vi "Configure TS Panel.vi"(8 "error in":errorcluster, 11 "DeepU Test Stand in":refnum<class "DeepU Test Stand.lvclass">) -> (0 "error out":errorcluster, 3 "DeepU Test Stand out":refnum<class "DeepU Test Stand.lvclass">)   [LabVIEW 2019, in "Test Stands.lvlib" / "DeepU Test Stand.lvclass"]
uses:
  DeepU Test Stand.lvclass
  C:/Users/wg/Documents/LV_Projects/test-stand/App/Generic Test Stand/Generic Test Stand.lvclass
  Generic Test Stand/Generic Test Stand.lvclass/Generic Test Stand.ctl
  DeepU Test Stand.lvclass/DeepU Test Stand.ctl
  Generic Test Stand/Generic Test Stand.lvclass
  Results/DeepU Results/DeepU Front Panel.vi
  Results/DeepU Results/DeepU Results.lvclass
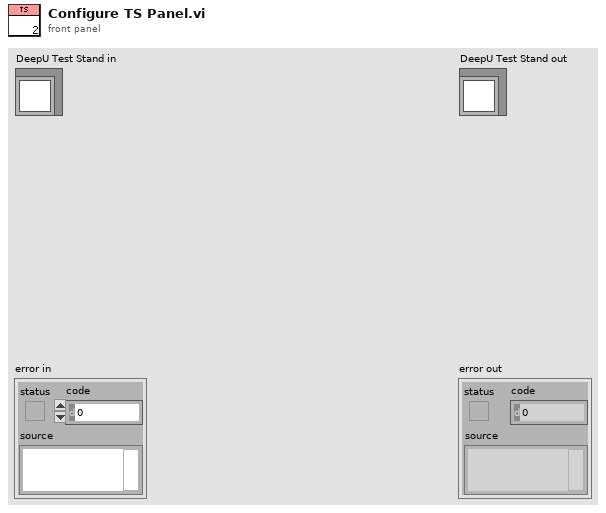
[diagram p1: front panel]
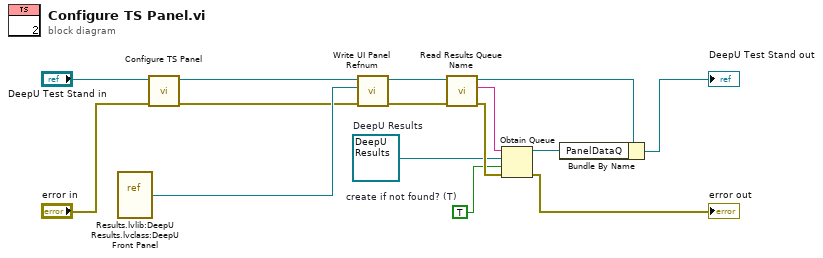
[diagram p0: block diagram]
diagram:
  w2 = refnum<class "DeepU Results.lvclass"> refnum  # DeepU Results
  w4 = TRUE  # create if not found? (T)
  n1 = vi-ref "Results.lvlib:DeepU Results.lvclass:DeepU Front Panel.vi"() -> (w15:refnum<vi>)
  n2 = call-parent "Configure TS Panel.vi"("error in (no error)"="error in", "Generic Test Stand in"="DeepU Test Stand in") -> ("error out"=w11:errorcluster, "Generic Test Stand out"=w13:refnum<class "DeepU Test Stand.lvclass">)  [unwired: 8 in]
  n3 = call "Write UI Panel Refnum.vi"("error in (no error)"=w11, "UI Panel Refnum"=w15, "Generic Test Stand in"=w13) -> ("error out"=w7:errorcluster, "Generic Test Stand out"=w10:refnum<class "DeepU Test Stand.lvclass">)  [unwired: 7 in]
  n4 = call "Read Results Queue Name.vi"("error in (no error)"=w7, "Generic Test Stand in"=w10) -> ("error out"=w5:errorcluster, "Results Queue Name"=w6:string, "Generic Test Stand out"=w9:refnum<class "DeepU Test Stand.lvclass">)  [unwired: 7 in]
  n5 = Obtain Queue(name (unnamed)=w6, element data type=w2, create if not found? (T)=w4, error in (no error)=w5) -> (queue out=w1:refnum<queue>, error out=→"error out":errorcluster)  [unwired: 1 in, 1 out]
  n6 = Bundle By Name(cluster=w9, "PanelDataQ"=w1) -> (→"DeepU Test Stand out":refnum<class "DeepU Test Stand.lvclass">)
